vi "Pose2d_Minus.vi"(9 "other TRANSFORM":T1 {"ROTATION"."SIN" format="%13.4f"; "ROTATION"."COS" format="%13.4f"; "ROTATION"."VALUE" format="%13.4f"; "TRANSLATION"."Y" format="%14.3f"; "TRANSLATION"."X" format="%14.3f"}, 11 "in POSE":T4 {"ROTATION"."SIN" format="%13.4f"; "ROTATION"."COS" format="%13.4f"; "ROTATION"."VALUE" format="%13.4f"; "TRANSLATION"."Y" format="%14.3f"; "TRANSLATION"."X" format="%14.3f"}) -> (3 "outTRANSFORM":T1={"TRANSLATION"={"X"=0.0, "Y"=0.0}, "ROTATION"={"VALUE"=0.0, "COS"=1.0, "SIN"=0.0}} {"ROTATION"."SIN" format="%13.4f"; "ROTATION"."COS" format="%13.4f"; "ROTATION"."VALUE" format="%13.4f"; "TRANSLATION"."Y" format="%14.3f"; "TRANSLATION"."X" format="%14.3f"})   [LabVIEW 2019, in "Trajectory_Library.lvlib"]
doc: "Returns the Transform2d that maps the one pose to another.\n\nParameter:\n - IN POSE - Current POSE data structure\n - OTHER POSE - The initial pose of the transformation.\n\nReturns:\n - OUT TRANSFORMATION - The transform that maps the other pose to the current pose."
uses:
  Trajectory_Library.lvlib
  POSE2D.ctl
  TRANSLATION2D.ctl
  ROTATION2D.ctl
  TRANSFORM2D.ctl
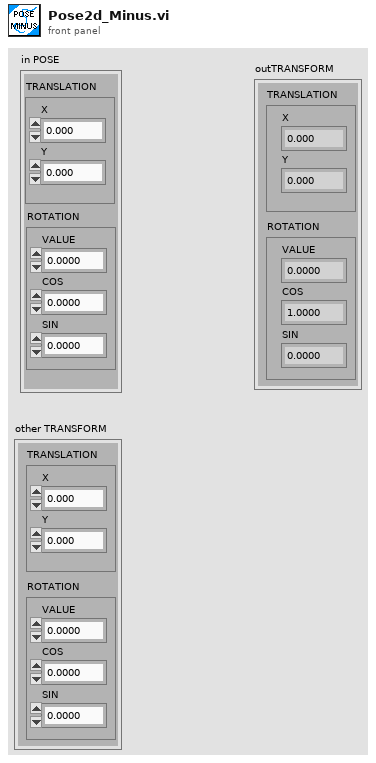
[diagram p1: front panel]
types:
  T1 = typedef "Trajectory_Library.lvlib/TRANSFORM2D.ctl" = cluster{"TRANSLATION":T2, "ROTATION":T3}
  T2 = typedef "Trajectory_Library.lvlib/TRANSLATION2D.ctl" = cluster{"X":dbl, "Y":dbl}
  T3 = typedef "Trajectory_Library.lvlib/ROTATION2D.ctl" = cluster{"VALUE":dbl, "COS":dbl, "SIN":dbl}
  T4 = typedef "Trajectory_Library.lvlib/POSE2D.ctl" = cluster{"TRANSLATION":T2, "ROTATION":T3}
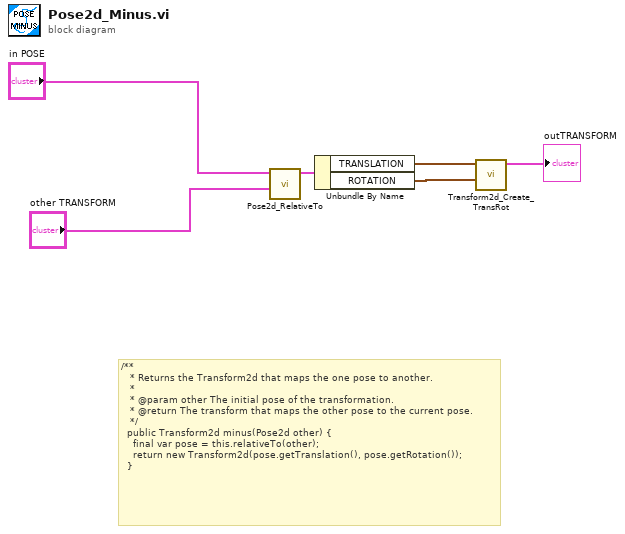
[diagram p0: block diagram]
diagram:
  # "/**\n   * Returns the Transform2d that maps the one pose to another.\n   *\n   * @param other The initial pose of the transformation.\n   * @return The transform that maps the other pose to the current pose.\n   */\n  public Transform2d minus(Pose2d other) {\n    final var pose = this.relativeTo(other);\n    return new Transform2d(pose.getTranslation(), pose.getRotation());\n  }"
  n1 = call "Pose2d_RelativeTo.vi"("other POSE"="other TRANSFORM", "in POSE"="in POSE") -> ("out POSE"=w4:T4)  [unwired: 9 in]
  n2 = Unbundle By Name(w4) -> ("TRANSLATION"=w3:T2, "ROTATION"=w2:T3)
  n3 = call "Transform2d_Create_TransRot.vi"("ROTATION"=w2, "TRANSLATION"=w3) -> ("TRANSFORM"=→"outTRANSFORM":T1)  [unwired: 9 in]
